vi "integralTrap.vi"(1 "n-int":i32 caption="number of points\nto integrate over", 2 "data Array":dbl[](array[numeric]), 3 "time Array":dbl[](array[numeric])) -> (0 "integral":dbl)   [LabVIEW 2024]
panel:
  out "Offset":i32
  out "Loop Run":i32
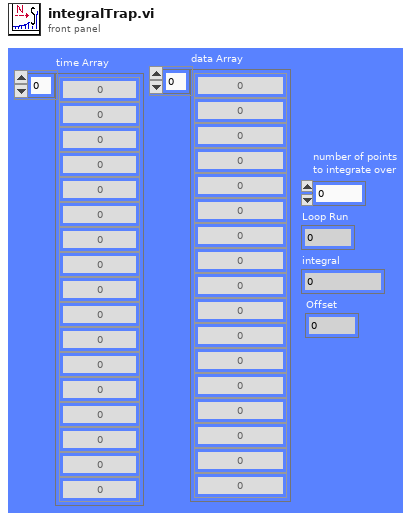
[diagram p1: front panel]
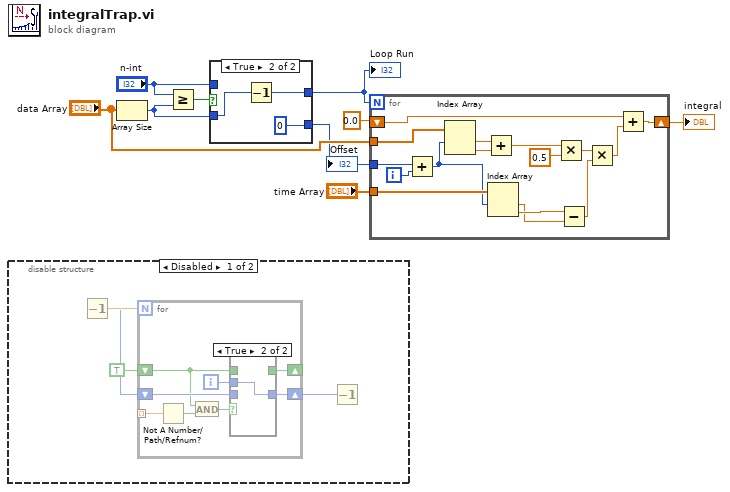
[diagram p0: block diagram]
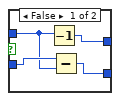
[diagram p2: hidden frame]
diagram:
  n1 = disable-structure shown="Disabled" {
    frame Disabled {
      n2 = Decrement(x=w10) -> (x-1=w11:dbl)
      n3 = for {
        N: w11 -> [_]
        tunnel: _ -> [w17] mode=indexing
        shift-right: [w20] -> _
        shift-left: TRUE -> [w14]
        shift-right: [w19] -> w12
        shift-left: [w18] -> w10
        i -> [w21]
        n4 = Not A Number/Path/Refnum?(number/path/refnum=w17) -> (NaN/Path/Refnum?=w15:bool)
        n5 = And(x=w14, y=w15) -> (x .and. y?=w16:bool)
        n6 = case shown="True" w16 {
          tunnel: w21 -> [_ w24]
          tunnel: [w22 _] -> w20
          tunnel: [w23 w24] -> w19
          tunnel: w18 -> [w23 _]
          tunnel: w14 -> [w22 _]
          frame False {
          }
          frame True {
          }
        }
      }
      n7 = Decrement(x=w12) -> ()  [unwired: 1 out]
    }
    frame Enabled {
    }
  }
  n8 = Array Size(array="data Array") -> (size(s)=w5:i32)
  n9 = Greater Or Equal?(x="n-int", y=w5) -> (x >= y?=w6:bool)
  n10 = case shown="True" w6 {
    tunnel: w5 -> [w27 w31]
    tunnel: [w28 w30] -> w4
    tunnel: [w25 0] -> w2
    tunnel: "n-int" -> [w26 _]
    frame False {
      n11 = Decrement(x=w26) -> (x-1=w28:i32)
      n12 = Subtract(x=w27, y=w26) -> (x-y=w25:i32)
    }
    frame True {
      n13 = Decrement(x=w31) -> (x-1=w30:i32)
    }
  }
  "Loop Run" <- w4
  "Offset" <- w2
  n14 = for {
    N: w4 -> [_]
    tunnel: "data Array" -> [w44]
    tunnel: "time Array" -> [w47]
    shift-right: [w45] -> w9
    shift-left: 0.0 -> [w46]
    tunnel: w2 -> [w36]
    i -> [w35]
    n15 = Add(x=w36, y=w35) -> (x+y=w34:i32)
    n16 = Index Array(array=w44, index #1=w34) -> (element #1=w38:dbl, element #2=w37:dbl)  [unwired: 1 in]
    n17 = Add(x=w38, y=w37) -> (x+y=w43:dbl)
    n18 = Index Array(array=w47, index #1=w34) -> (element #1=w32:dbl, element #2=w33:dbl)  [unwired: 1 in]
    n19 = Multiply(x=w43, y=0.5) -> (x*y=w40:dbl)
    n20 = Subtract(x=w33, y=w32) -> (x-y=w41:dbl)
    n21 = Multiply(x=w40, y=w41) -> (x*y=w39:dbl)
    n22 = Add(x=w46, y=w39) -> (x+y=w45:dbl)
  }
  "integral" <- w9
